vi "外观 1.vi"(0 "Data In":T5 caption="数据输入", 2 "Display State In":T3 caption="显示状态输入", 3 "Container State":T4 caption="容器状态") -> (6 "Data Out":T5 caption="数据输出", 7 "Display State Out":T3 caption="显示状态输出", 8 "Action":T2 caption="动作")   [LabVIEW 2016, in "氨氮曲线模型.xctl"]
uses:
  <vilib>/_xctls/Container State.ctl
  <vilib>/_xctls/Action.ctl
  <vilib>/_xctls/XControlSupport.lvlib
  <vilib>/Utility/config.llb/NI_LVConfig.lvlib
panel:
  in  "曲线模型":T1={"标液浓度1"=0.0, "样品1 F0"=0.0, "样品1 F1"=0.0, "测量吸光度1"=0.0, "样品1启用"=FALSE, "标液浓度2"=0.0, "样品2 F0"=0.0, "样品2 F1"=0.0, "测量吸光度2"=0.0, "样品2启用"=FALSE, "标液浓度3"=0.0, "样品3 F0"=0.0, "样品3 F1"=0.0, "测量吸光度3"=0.0, "样品3启用"=FALSE, "标液浓度4"=0.0, "样品4 F0"=0.0, "样品4 F1"=0.0, "测量吸光度4"=0.0, "样品4启用"=FALSE, "标液浓度5"=0.0, "样品5 F0"=0.0, "样品5 F1"=0.0, "测量吸光度5"=0.0, "样品5启用"=FALSE, "模型"=enum."线性", "method"=0, "精度"=4.0, "XY图"=[], "拟合公式"="", "r^2"=0.0} {"method" items=["最小二乘", "最小绝对残差", "Bisquare"]; "r^2" format="%.7g"}
  # "标液浓度"
  # "F0"
  # "F1"
  # "吸光值显示"
  # "样品一"
  # "辅\n助\n计\n算\n区"
  # "样品二"
  # "样品三"
  # "样品四"
  # "样品五"
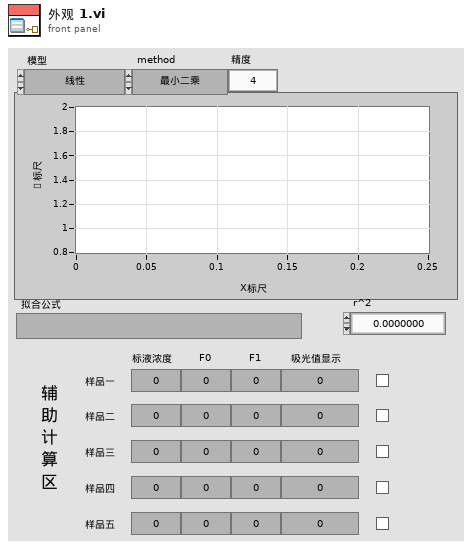
[diagram p1: front panel]
types:
  T1 = cluster{"标液浓度1":dbl, "样品1 F0":dbl, "样品1 F1":dbl, "测量吸光度1":dbl, "样品1启用":bool, "标液浓度2":dbl, "样品2 F0":dbl, "样品2 F1":dbl, "测量吸光度2":dbl, "样品2启用":bool, "标液浓度3":dbl, "样品3 F0":dbl, "样品3 F1":dbl, "测量吸光度3":dbl, "样品3启用":bool, "标液浓度4":dbl, "样品4 F0":dbl, "样品4 F1":dbl, "测量吸光度4":dbl, "样品4启用":bool, "标液浓度5":dbl, "样品5 F0":dbl, "样品5 F1":dbl, "测量吸光度5":dbl, "样品5启用":bool, "模型":enum32{"线性", "多项式"}, "method":u16, "精度":dbl, "XY图":cluster{"X Values":dbl[], "Y Values":dbl[]}[], "拟合公式":string, "r^2":dbl}
  T2 = typedef "XControlSupport.lvlib/Action.ctl" = cluster{"Data Changed?":bool, "State Changed?":bool, "Action Name":string}
  T3 = typedef "氨氮曲线模型.xctl/状态 1.ctl" = cluster{"调用模块名称":string}
  T4 = typedef "XControlSupport.lvlib/Container State.ctl" = cluster{"Indicator?":bool, "Run Mode?":bool, " Refnum":refnum<vi>}
  T5 = typedef "氨氮曲线模型.xctl/数据 1.ctl" = cluster{"X^2":dbl, "X":dbl, "B":dbl}
  T6 = typedef "NI_LVConfig.lvlib/Config Data RefNum.ctl" = refnum<k1>
  T7 = cluster{"Polynomial Coefficients[0]":dbl, "Polynomial Coefficients[1]":dbl, "Polynomial Coefficients[2]":dbl}
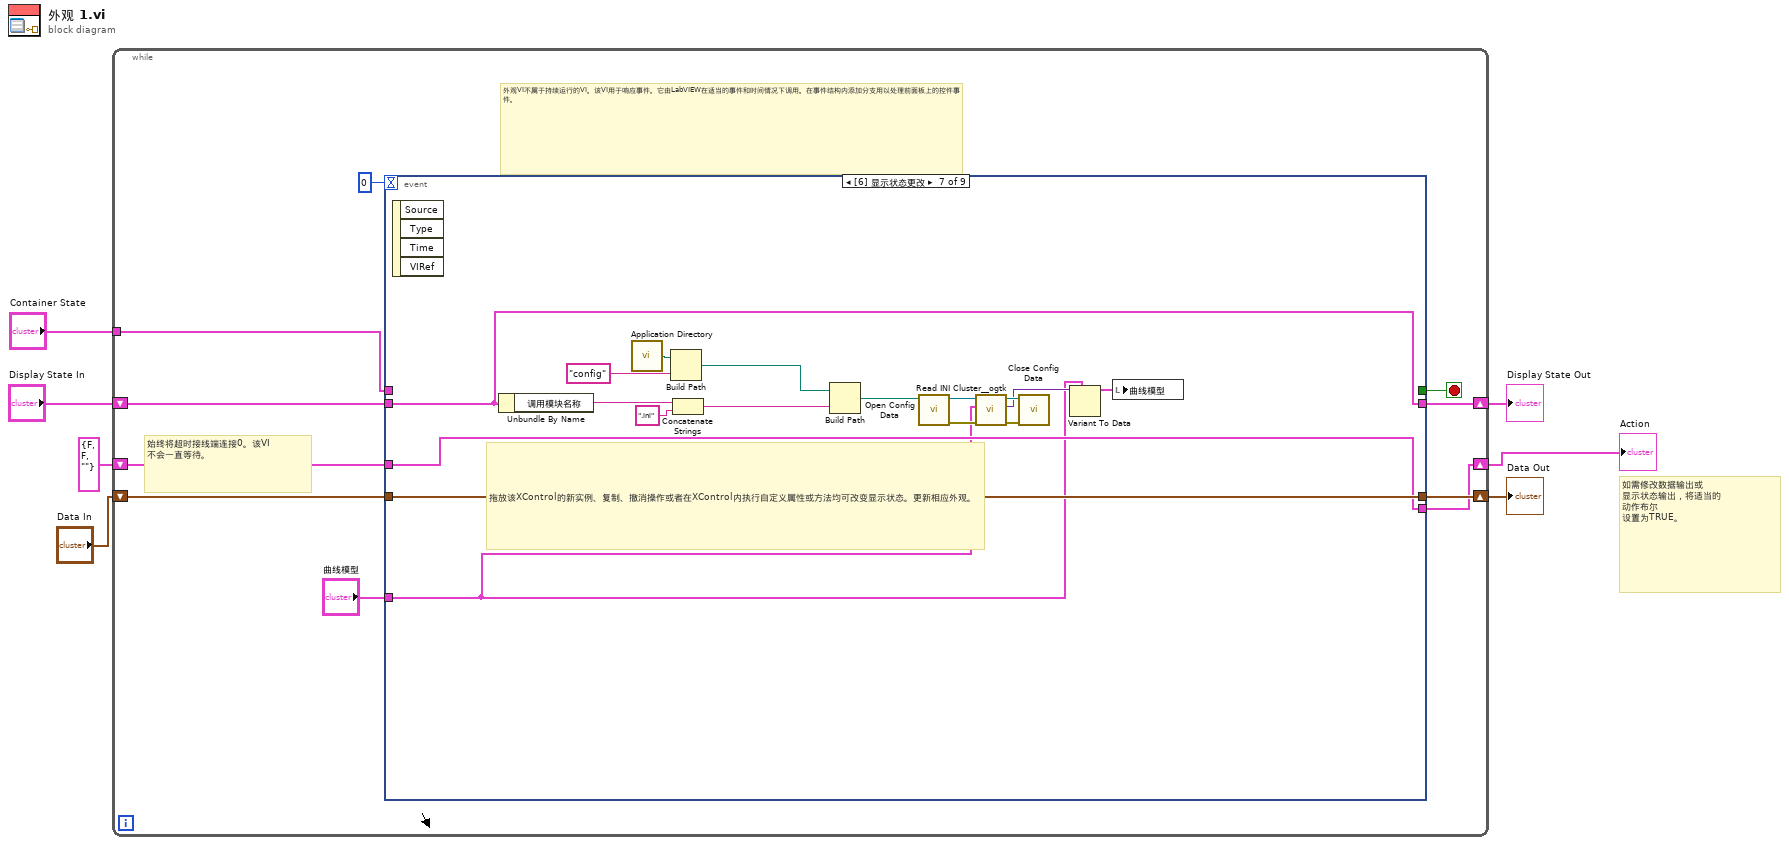
[diagram p0: block diagram]
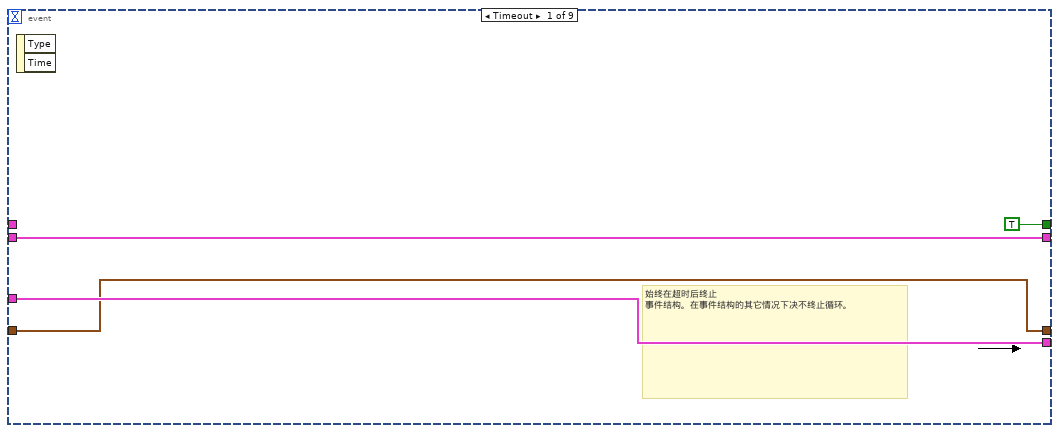
[diagram p2: hidden frame]
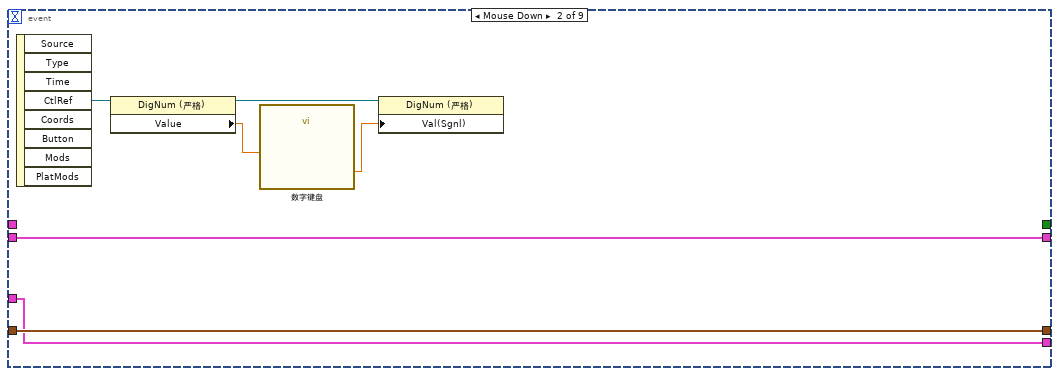
[diagram p3: hidden frame]
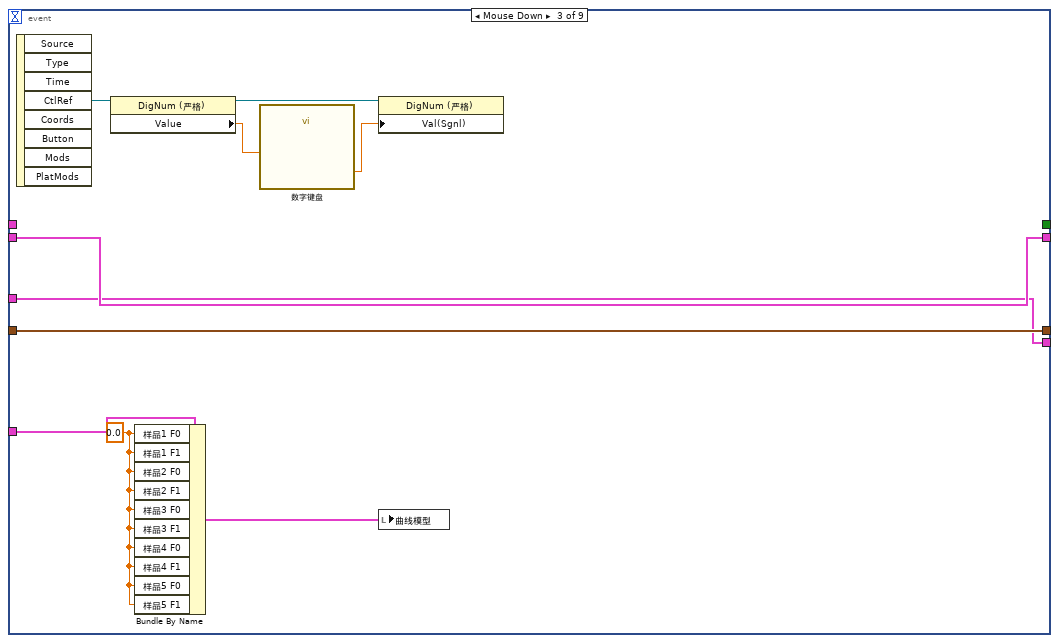
[diagram p4: hidden frame]
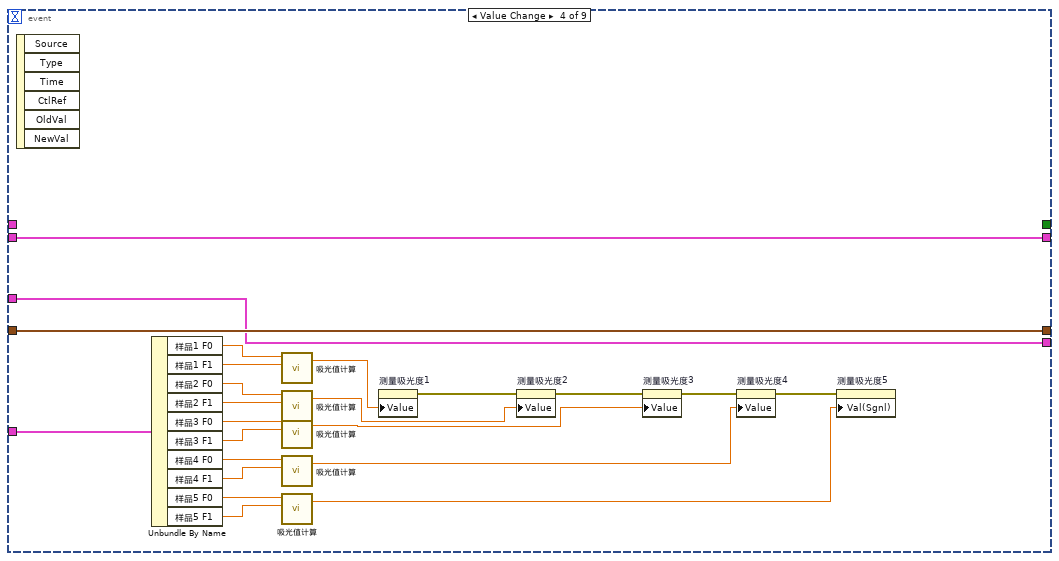
[diagram p5: hidden frame]
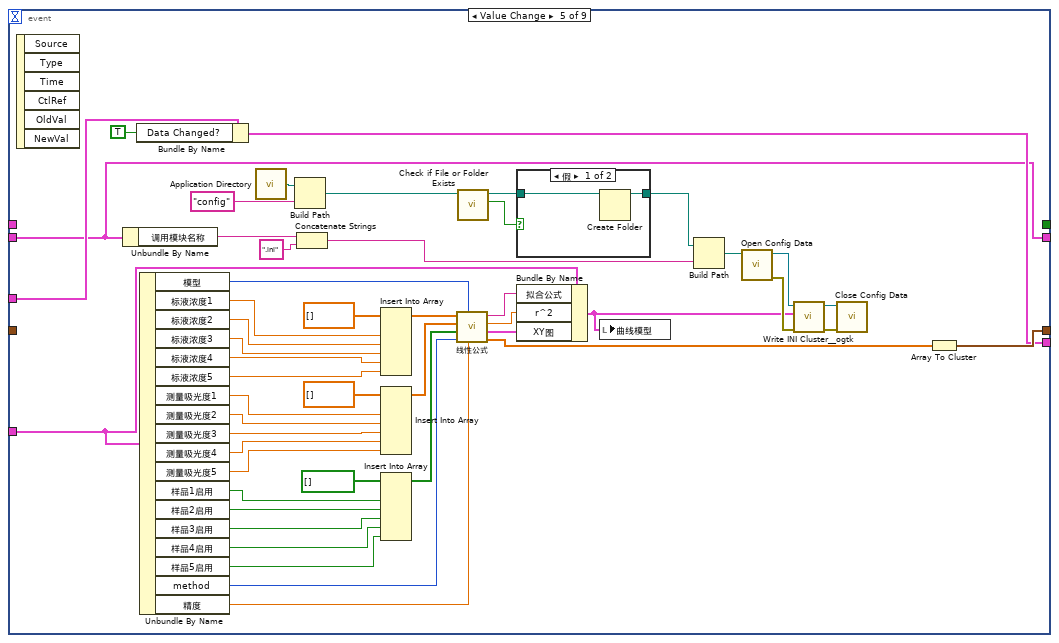
[diagram p6: hidden frame]
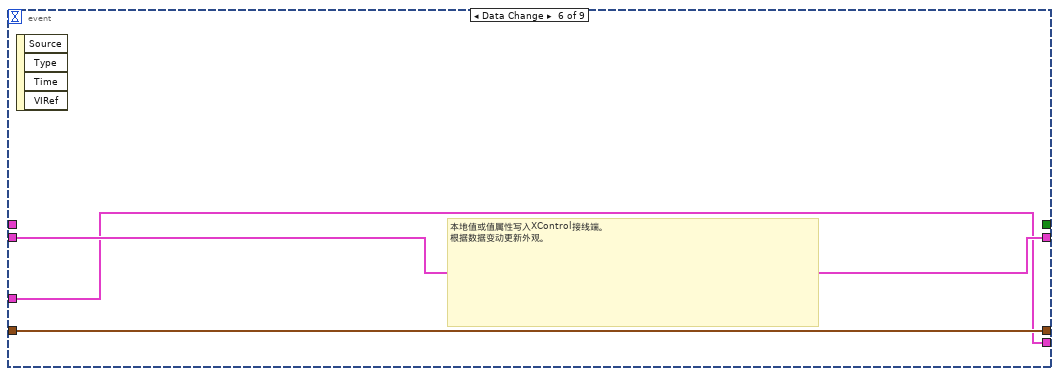
[diagram p8: hidden frame]
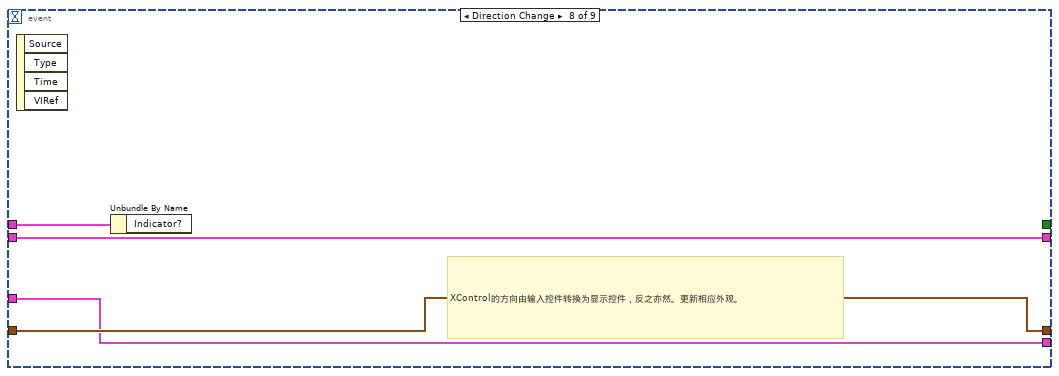
[diagram p9: hidden frame]
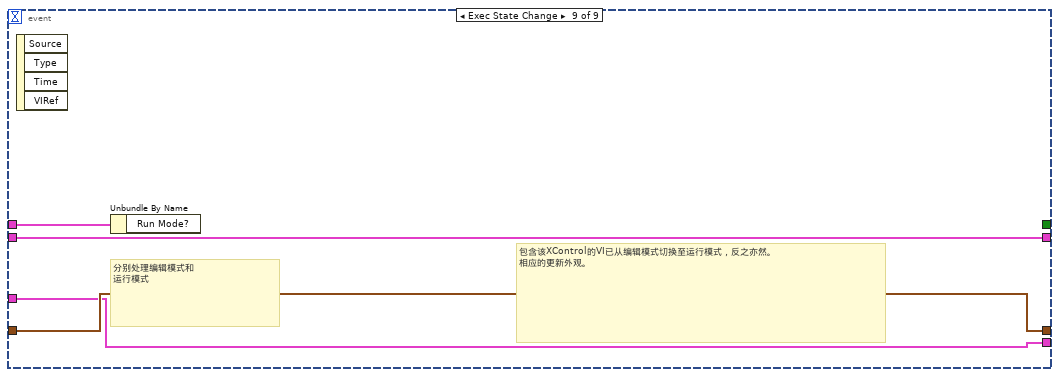
[diagram p10: hidden frame]
diagram:
  # "如需修改数据输出或\n显示状态输出，将适当的\n动作布尔\n设置为TRUE。"
  n1 = while {
    shift-right: [w16] -> w4
    shift-left: "Display State In" -> [w17]
    tunnel: "Container State" -> [w13]
    shift-right: [w11] -> w7
    shift-left: "Data In" -> [w12]
    shift-right: [w9] -> w2
    shift-left: T2 {"Data Changed?"=FALSE, "State Changed?"=FALSE, "Action Name"=""} ("Action") -> [w10]
    stop <- w15 stop-if-true
    # "外观VI不属于持续运行的VI。该VI用于响应事件。它由LabVIEW在适当的事件和时间情况下调用。在事件结构内添加分支用以处理前面板上的控件事件。"
    # "始终将超时接线端连接0。该VI\n不会一直等待。"
    n2 = event shown="[6] 显示状态更改" {
      selector: _ -> [_ _ _ _ _ _ _ _ _]
      dyn-events: _ -> [_ _ _ _ _ _ _ _ _]
      timeout: 0 -> [_ _ _ _ _ _ _ _ _]
      tunnel: w17 -> [w19 w28 w38 w61 w67 w115 w126 w136 w140]
      tunnel: [w19 w28 w38 w61 w67 w115 w126 w136 w140] -> w16
      tunnel: [TRUE _ _ _ _ _ _ _ _] -> w15
      tunnel: w13 -> [_ _ _ _ _ _ _ w137 w141]
      tunnel: w12 -> [w18 w27 w37 w60 _ w116 w133 w135 w139]
      tunnel: [w18 w27 w37 w60 w81 w116 w133 w135 w139] -> w11
      tunnel: [w20 w26 w36 w59 w78 w114 w127 w134 w138] -> w9
      tunnel: w10 -> [w20 w26 w36 w59 w80 w114 w127 w134 w138]
      tunnel: "曲线模型" -> [_ _ w31 w48 w86 _ w118 _ _]
      event Timeout {
        # "始终在超时后终止\n事件结构。在事件结构的其它情况下决不终止循环。"
        n3 = event-data() -> ()  [unwired: 1 in, 2 out]
      }
      event "曲线模型.标液浓度1", "曲线模型.样品1 F0", "曲线模型.样品1 F1", "曲线模型.标液浓度2", "曲线模型.样品2 F0", "曲线模型.样品2 F1", "曲线模型.标液浓度3", "曲线模型.样品3 F0", "曲线模型.样品3 F1", "曲线模型.标液浓度4", "曲线模型.样品4 F0", "曲线模型.样品4 F1", "曲线模型.标液浓度5", "曲线模型.样品5 F0", "曲线模型.样品5 F1", "曲线模型.精度": Mouse Down {
        n4 = event-data() -> ("CtlRef"=w25:refnum<vi>)  [unwired: 1 in, 7 out]
        n5 = property class="DigNum (严格)"(reference=w25) -> (reference out=w22:refnum<vi>, "Value"=w24:dbl)  [unwired: 1 in, 1 out]
        n6 = call "数字键盘.vi"("OldNumber"=w24) -> ("NewNumber"=w23:dbl)
        n7 = property class="DigNum (严格)"(reference=w22, "Val(Sgnl)"=w23) -> ()  [unwired: 1 in, 2 out]
      }
      event "曲线模型.测量吸光度1", "曲线模型.测量吸光度2", "曲线模型.测量吸光度3", "曲线模型.测量吸光度4", "曲线模型.测量吸光度5": Mouse Down {
        w30 = 0.0 ("测量吸光度1")
        n8 = event-data() -> ("CtlRef"=w35:refnum<vi>)  [unwired: 1 in, 7 out]
        n9 = property class="DigNum (严格)"(reference=w35) -> (reference out=w32:refnum<vi>, "Value"=w34:dbl)  [unwired: 1 in, 1 out]
        n10 = Bundle By Name(cluster=w31, "样品1 F0"=w30, "样品1 F1"=w30, "样品2 F0"=w30, "样品2 F1"=w30, "样品3 F0"=w30, "样品3 F1"=w30, "样品4 F0"=w30, "样品4 F1"=w30, "样品5 F0"=w30, "样品5 F1"=w30) -> (w29:T1)
        n11 = call "数字键盘.vi"("OldNumber"=w34) -> ("NewNumber"=w33:dbl)
        n12 = property class="DigNum (严格)"(reference=w32, "Val(Sgnl)"=w33) -> ()  [unwired: 1 in, 2 out]
        n13 = local write "曲线模型"(w29) -> ()
      }
      event "曲线模型.样品1 F0", "曲线模型.样品1 F1", "曲线模型.样品2 F0", "曲线模型.样品2 F1", "曲线模型.样品3 F0", "曲线模型.样品3 F1", "曲线模型.样品4 F0", "曲线模型.样品4 F1", "曲线模型.样品5 F0", "曲线模型.样品5 F1": Value Change {
        n14 = event-data() -> ()  [unwired: 1 in, 6 out]
        n15 = Unbundle By Name(w48) -> ("样品1 F0"=w58:dbl, "样品1 F1"=w57:dbl, "样品2 F0"=w49:dbl, "样品2 F1"=w50:dbl, "样品3 F0"=w51:dbl, "样品3 F1"=w52:dbl, "样品4 F0"=w53:dbl, "样品4 F1"=w54:dbl, "样品5 F0"=w55:dbl, "样品5 F1"=w56:dbl)
        n16 = call "吸光值计算.vi"("F1"=w57, "F0"=w58) -> ("测量吸光度"=w43:dbl)  [unwired: 3 in]
        n17 = call "吸光值计算.vi"("F1"=w50, "F0"=w49) -> ("测量吸光度"=w42:dbl)  [unwired: 3 in]
        n18 = call "吸光值计算.vi"("F1"=w52, "F0"=w51) -> ("测量吸光度"=w41:dbl)  [unwired: 3 in]
        n19 = call "吸光值计算.vi"("F1"=w54, "F0"=w53) -> ("测量吸光度"=w40:dbl)  [unwired: 3 in]
        n20 = call "吸光值计算.vi"("F1"=w56, "F0"=w55) -> ("测量吸光度"=w39:dbl)  [unwired: 3 in]
        n21 = property on="测量吸光度1" class="DigNum (严格)"("Value"=w43) -> (error out=w47:errorcluster)  [unwired: 2 in, 1 out]
        n22 = property on="测量吸光度2" class="DigNum (严格)"(error in=w47, "Value"=w42) -> (error out=w46:errorcluster)  [unwired: 1 in, 1 out]
        n23 = property on="测量吸光度3" class="DigNum (严格)"(error in=w46, "Value"=w41) -> (error out=w45:errorcluster)  [unwired: 1 in, 1 out]
        n24 = property on="测量吸光度4" class="DigNum (严格)"(error in=w45, "Value"=w40) -> (error out=w44:errorcluster)  [unwired: 1 in, 1 out]
        n25 = property on="测量吸光度5" class="DigNum (严格)"(error in=w44, "Val(Sgnl)"=w39) -> ()  [unwired: 1 in, 2 out]
      }
      event "曲线模型.标液浓度1", "曲线模型.测量吸光度1", "曲线模型.标液浓度2", "曲线模型.测量吸光度2", "曲线模型.样品1启用", "曲线模型.样品2启用", "曲线模型.标液浓度3", "曲线模型.测量吸光度3", "曲线模型.样品3启用", "曲线模型.标液浓度4", "曲线模型.测量吸光度4", "曲线模型.样品4启用", "曲线模型.标液浓度5", "曲线模型.测量吸光度5", "曲线模型.样品5启用", "曲线模型.模型", "曲线模型.method", "曲线模型.精度": Value Change {
        n26 = event-data() -> ()  [unwired: 1 in, 6 out]
        n27 = Unbundle By Name(w67) -> ("调用模块名称"=w62:string)
        n28 = Bundle By Name(cluster=w80, "Data Changed?"=TRUE) -> (w78:T2)
        n29 = Unbundle By Name(w86) -> ("模型"=w110:enum32{"线性", "多项式"}, "标液浓度1"=w106:dbl, "标液浓度2"=w105:dbl, "标液浓度3"=w104:dbl, "标液浓度4"=w103:dbl, "标液浓度5"=w102:dbl, "测量吸光度1"=w99:dbl, "测量吸光度2"=w98:dbl, "测量吸光度3"=w97:dbl, "测量吸光度4"=w96:dbl, "测量吸光度5"=w95:dbl, "样品1启用"=w92:bool, "样品2启用"=w91:bool, "样品3启用"=w90:bool, "样品4启用"=w89:bool, "样品5启用"=w88:bool, "method"=w109:u16, "精度"=w108:dbl)
        n30 = call <vilib>:"Application Directory.vi"() -> ("Application Directory"=w72:path)
        n31 = Build Path(base path=w72, name or relative path="config" ("名称或相对路径")) -> (appended path=w70:path)
        n32 = Concatenate Strings(w62, ".ini" ("字符串")) -> (w66:string)
        n33 = Insert Into Array(array=dbl[] [] ("标液浓度"), new element #1=w106, new element #2=w105, new element #3=w104, new element #4=w103, new element #5=w102) -> (w101:dbl[])  [unwired: 1 in]
        n34 = Insert Into Array(array=dbl[] [] ("标液浓度"), new element #1=w99, new element #2=w98, new element #3=w97, new element #4=w96, new element #5=w95) -> (w94:dbl[])  [unwired: 1 in]
        n35 = Insert Into Array(array=bool[] [] ("启用"), new element #1=w92, new element #2=w91, new element #3=w90, new element #4=w89, new element #5=w88) -> (w87:bool[])  [unwired: 1 in]
        n36 = call "线性公式.vi"("精度"=w108, "模型"=w110, "method"=w109, "启用"=w87, "监测浓度"=w94, "标液浓度"=w101) -> ("Polynomial Coefficients"=w82:dbl[], "XY图"=w83:cluster{"X Values":dbl[], "Y Values":dbl[]}[], "r^2"=w84:dbl, "拟合方程"=w85:string)  [unwired: 2 in]
        n37 = call <vilib>:"Check if File or Folder Exists.vi"("path"=w70) -> ("file or folder exists?"=w69:bool, "dup path"=w68:path)  [unwired: 8 in, 1 out]
        n38 = case shown="假" w69 {
          tunnel: w68 -> [w112 w113]
          tunnel: [w111 w113] -> w64
          frame False {
            n39 = Create Folder(path (use dialog)=w112) -> (created path=w111:path)  [unwired: 2 in, 2 out]
          }
          frame True {
          }
        }
        n40 = Bundle By Name(cluster=w86, "拟合公式"=w85, "r^2"=w84, "XY图"=w83) -> (w75:T1)
        n41 = local write "曲线模型"(w75) -> ()
        n42 = Build Path(base path=w64, name or relative path=w66) -> (appended path=w63:path)
        n43 = call <vilib>:"Open Config Data.vi"("configuration file path"=w63) -> ("error out"=w76:errorcluster, "refnum"=w77:T6)  [unwired: 8 in, 1 out]
        n44 = call <userlib>:"Write INI Cluster__ogtk.vi"("error in (no error)"=w76, "INI Fomatted Cluster"=w75, "refnum"=w77) -> ("error out"=w73:errorcluster, "dup refnum"=w74:T6)  [unwired: 7 in]
        n45 = call <vilib>:"Close Config Data.vi"("error in (no error)"=w73, "refnum"=w74) -> ()  [unwired: 8 in, 2 out]
        n46 = Array To Cluster(array=w82) -> (cluster=w81:T7)
      }
      event Data Change {
        # "本地值或值属性写入XControl接线端。\n根据数据变动更新外观。"
        n47 = event-data() -> ()  [unwired: 1 in, 4 out]
      }
      event Display State Change {
        # "拖放该XControl的新实例、复制、撤消操作或者在XControl内执行自定义属性或方法均可改变显示状态。更新相应外观。"
        n48 = event-data() -> ()  [unwired: 1 in, 4 out]
        n49 = Unbundle By Name(w126) -> ("调用模块名称"=w122:string)
        n50 = call <vilib>:"Application Directory.vi"() -> ("Application Directory"=w125:path)
        n51 = Build Path(base path=w125, name or relative path="config" ("名称或相对路径")) -> (appended path=w123:path)
        n52 = Concatenate Strings(w122, ".ini" ("字符串")) -> (w120:string)
        n53 = Build Path(base path=w123, name or relative path=w120) -> (appended path=w128:path)
        n54 = call <vilib>:"Open Config Data.vi"("configuration file path"=w128) -> ("error out"=w131:errorcluster, "refnum"=w132:T6)  [unwired: 8 in, 1 out]
        n55 = call <userlib>:"Read INI Cluster__ogtk.vi"("error in (no error)"=w131, "INI Fomatted Cluster Type"=w118, "refnum"=w132) -> ("error out"=w129:errorcluster, "INI Fomatted Cluster"=w119:variant, "dup refnum"=w130:T6)  [unwired: 4 in, 2 out]
        n56 = call <vilib>:"Close Config Data.vi"("error in (no error)"=w129, "refnum"=w130) -> ()  [unwired: 8 in, 2 out]
        n57 = Variant To Data(type=w118, Variant=w119) -> (data=w117:T1)  [unwired: 1 in, 1 out]
        n58 = local write "曲线模型"(w117) -> ()
      }
      event Direction Change {
        # "XControl的方向由输入控件转换为显示控件，反之亦然。更新相应外观。"
        n59 = event-data() -> ()  [unwired: 1 in, 4 out]
        n60 = Unbundle By Name(w137) -> ()  [unwired: 1 out]
      }
      event Exec State Change {
        # "包含该XControl的VI已从编辑模式切换至运行模式，反之亦然。\n相应的更新外观。"
        # "分别处理编辑模式和\n运行模式"
        n61 = event-data() -> ()  [unwired: 1 in, 4 out]
        n62 = Unbundle By Name(w141) -> ()  [unwired: 1 out]
      }
    }
  }
  "Display State Out" <- w4
  "Data Out" <- w7
  "Action" <- w2
